vi "Close.vi"(8 "error in":errorcluster, 11 "Handler in":refnum<class "Handler.lvclass">) -> (0 "error out":errorcluster, 3 "Handler out":refnum<class "Handler.lvclass">)   [LabVIEW 2016, in "hse-logger.lvlib" / "Handler.lvclass"]
doc: "Tidy up any resources used by the handler. This method should be called when the ``Logger`` gets closed or the handler is removed from the ``Logger``.\n\nThis method is the implementation of the base-class and does nothing."
uses:
  Handler.lvclass
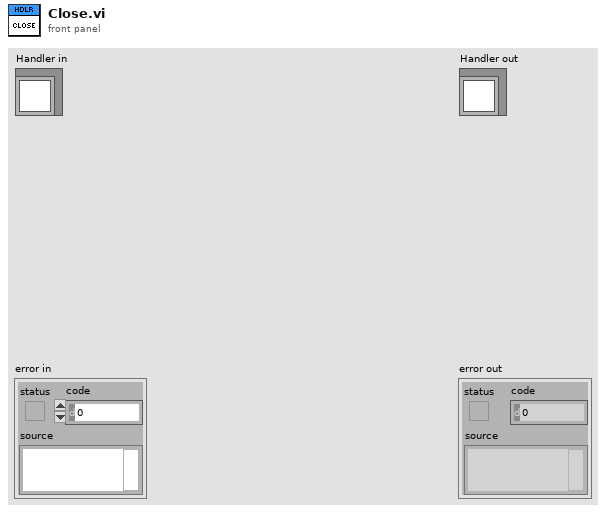
[diagram p1: front panel]
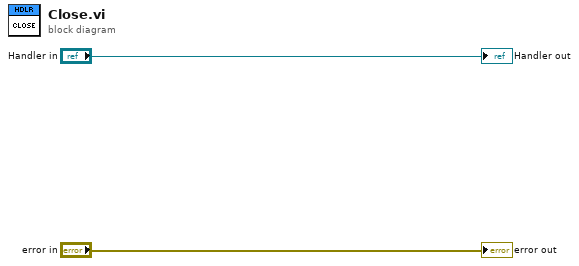
[diagram p0: block diagram]
diagram:
  "error out" <- "error in"
  "Handler out" <- "Handler in"
